vi "Chart[Template].DVRtoRef.vi"(10 "Ref":T1) -> (2 "Ref":u32 format="%08x")   [LabVIEW 2020, in "DisplayWaveform.lvlib" / "DisplayWaveforms.lvclass"]
doc: "JKI State Machine Objects (SMO) 1.0.0.5\nJKI - JKI\nCopyright (c) 2016, JKI"
uses:
  DisplayWaveforms.lvclass
  Typedefs/PrivateData--Ref.ctl
  Typedefs/PrivateData--Cluster.ctl
  Typedefs/PublicEvents--Cluster.ctl
  Typedefs/ProtectedEvents--Cluster.ctl
  Controller/TypeDefs/ChartParamsCluster.ctl
  Typedefs/Dependencies--Cluster.ctl
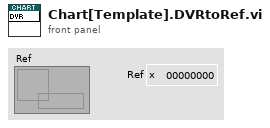
[diagram p1: front panel]
types:
  T1 = typedef "DisplayWaveform.lvlib/DisplayWaveforms.lvclass/PrivateData--Ref.ctl" = refnum<data-value>
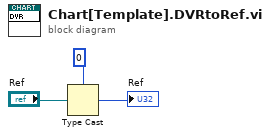
[diagram p0: block diagram]
diagram:
  n1 = Type Cast(type=u32 0 ("Ref"), x="Ref") -> (*(type *) &x=→"Ref":u32)
